vi "Test_simple-write.vi"() -> ()   [LabVIEW 2014]
uses:
  <vilib>/addons/h5labview2/file/H5Fmode.ctl
  <vilib>/addons/h5labview2/base/lib_path.vi
  <vilib>/addons/h5labview2/base/H5Equery.vi
  <vilib>/addons/h5labview2/dataset/H5Dwrite.llb/H5Dwrite.xnode
  <vilib>/addons/h5labview2/base/hid_t.ctl
  <vilib>/addons/h5labview2/attrib/H5Awrite.llb/H5Awrite.xnode
  <vilib>/addons/h5labview2/file/H5F.lvlib
  <vilib>/addons/h5labview2/group/H5G.lvlib
panel:
  out "Average time to write (ms)":dbl
  in  "Number of iterations":i32
  out "Time to Write (ms)":i32
  out "error out":errorcluster
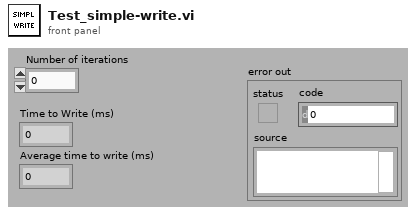
[diagram p1: front panel]
types:
  T1 = typedef "H5F.lvlib/H5Fmode.ctl" = enum16{"read-only", "read-write", "overwrite", "create new", "open or create"}
  T2 = typedef "hid_t.ctl" = i32
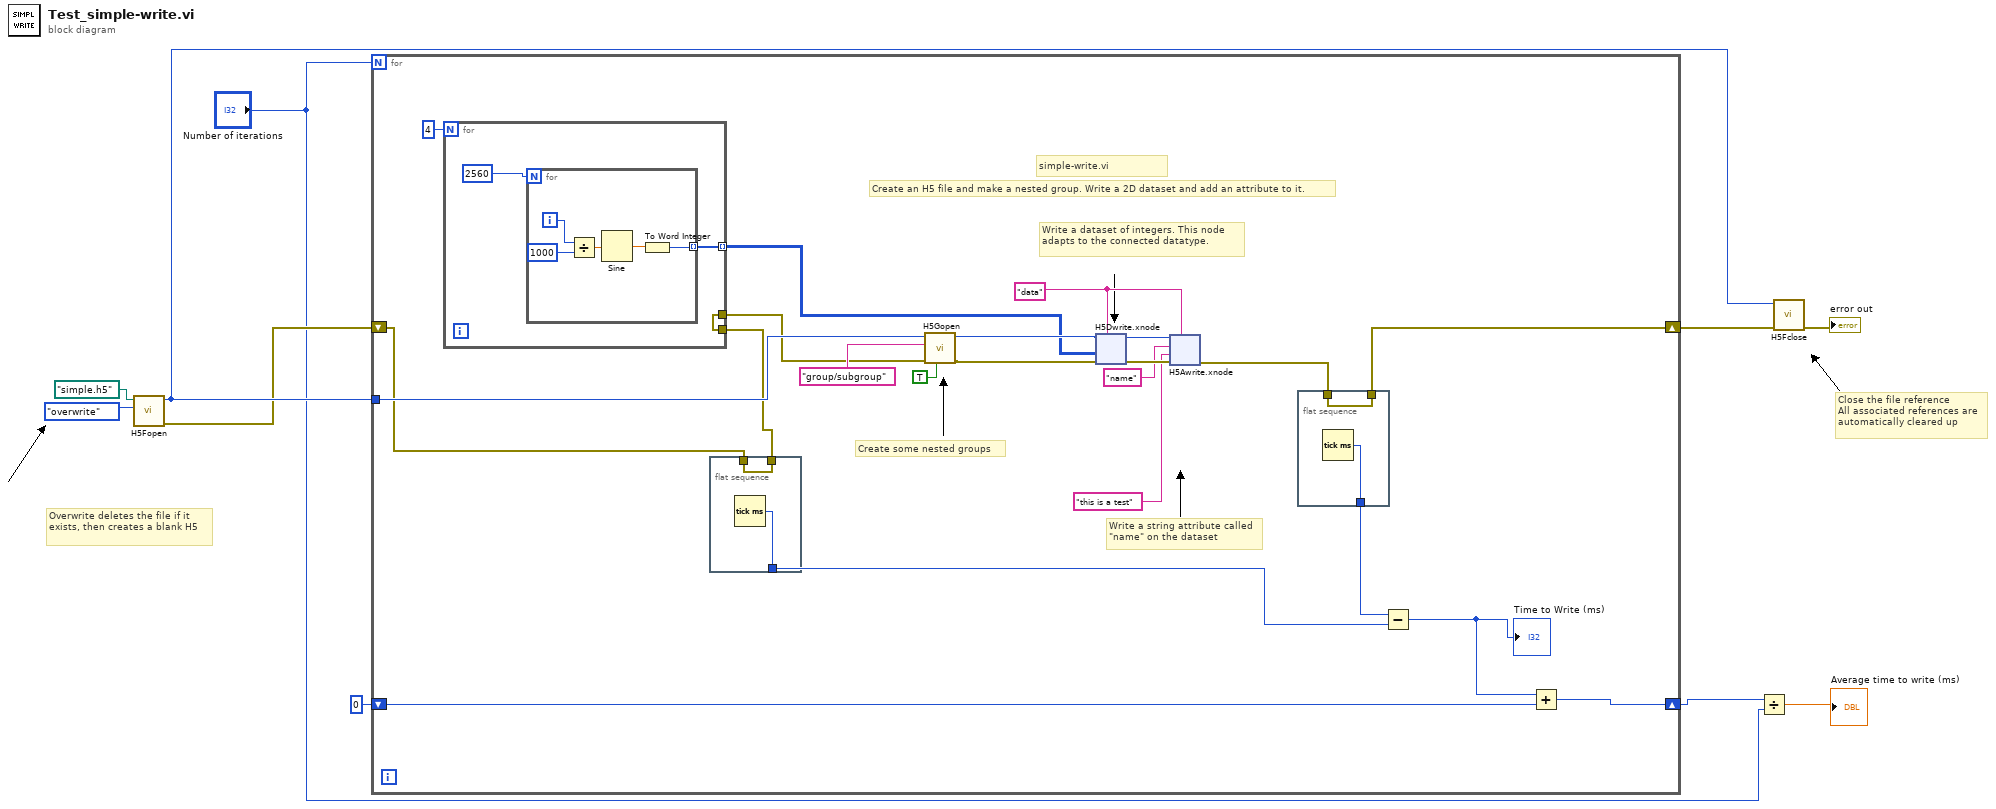
[diagram p0: block diagram]
diagram:
  # "Overwrite deletes the file if it exists, then creates a blank H5"
  # "Close the file reference\nAll associated references are\nautomatically cleared up"
  n1 = call <vilib>:"H5Fopen.vi"("mode (read-only)"=H5Fmode."overwrite" ("mode"), "path"=path "simple.h5" ("name or relative path")) -> ("error out"=w5:errorcluster, "ref out"=w9:T2)  [unwired: 8 in]
  n2 = for {
    N: "Number of iterations" -> [_]
    tunnel: w9 -> [w32]
    shift-right: [w21] -> w6
    shift-left: w5 -> [w14]
    shift-right: [w13] -> w2
    shift-left: u32 0 -> [w11]
    w25 = "data" ("name")
    # "Create an H5 file and make a nested group. Write a 2D dataset and add an attribute to it."
    # "simple-write.vi"
    # "Write a string attribute called\n\"name\" on the dataset"
    # "Write a dataset of integers. This node adapts to the connected datatype."
    # "Create some nested groups"
    n3 = for {
      N: 4 -> [_]
      tunnel: [w38] -> w23 mode=indexing
      tunnel: w16 -> [w37]
      tunnel: [w37] -> w15
      n4 = for {
        N: 2560 -> [_]
        tunnel: [w40] -> w38 mode=indexing
        i -> [w43]
        n5 = Divide(x=w43, y=1000) -> (x/y=w44:dbl)
        n6 = Sine(x=w44) -> (sin(x)=w41:dbl)
        n7 = To Word Integer(number=w41) -> (16bit integer=w40:i16)
      }
    }
    n8 = flat-sequence {
      tunnel: [w36] -> w19
      tunnel: w14 -> [w35]
      tunnel: [w35] -> w16
      frame #0 {
        n9 = Tick Count (ms)() -> (millisecond timer value=w36:u32)
      }
    }
    n10 = call <vilib>:"H5Gopen.vi"("create? (F)"=TRUE, "error in (no error)"=w15, "name"="group/subgroup", "ref in"=w32) -> ("error out"=w17:errorcluster, "group out"=w24:T2)  [unwired: 6 in]
    n11 = xnode "H5Dwrite.xnode"("dataset name"=w25, "error in (no error)"=w17, "data"=w23, "ref in"=w24) -> ("error out"=w28:errorcluster, "ref out"=w29:T2)  [unwired: 3 in, 1 out]
    n12 = xnode "H5Awrite.xnode"("object name"=w25, "error in (no error)"=w28, "data"="this is a test" ("name"), "attrib name"="name" ("name"), "ref in"=w29) -> ("error out"=w22:errorcluster)  [unwired: 2 in, 2 out]
    n13 = flat-sequence {
      tunnel: w22 -> [w34]
      tunnel: [w34] -> w21
      tunnel: [w33] -> w20
      frame #0 {
        n14 = Tick Count (ms)() -> (millisecond timer value=w33:u32)
      }
    }
    n15 = Subtract(x=w20, y=w19) -> (x-y=w12:u32)
    "Time to Write (ms)" <- w12
    n16 = Add(x=w12, y=w11) -> (x+y=w13:u32)
  }
  n17 = Divide(x=w2, y="Number of iterations") -> (x/y=→"Average time to write (ms)":dbl)
  n18 = call <vilib>:"H5Fclose.vi"("error in (no error)"=w6, "ref"=w9) -> ("error out"=→"error out":errorcluster)  [unwired: 9 in]
